vi "Get Root Elements.vi"(8 "error in (no error)":errorcluster, 11 "xml structure in":T1) -> (0 "error out":errorcluster, 1 "tag indices":i32[](array[numeric]), 2 "tag names":string[](array[string]), 3 "xml structure out":T1)   [LabVIEW 2011]
uses:
  XML Structure - Cluster.ctl
  XML Tag Type - Enum.ctl
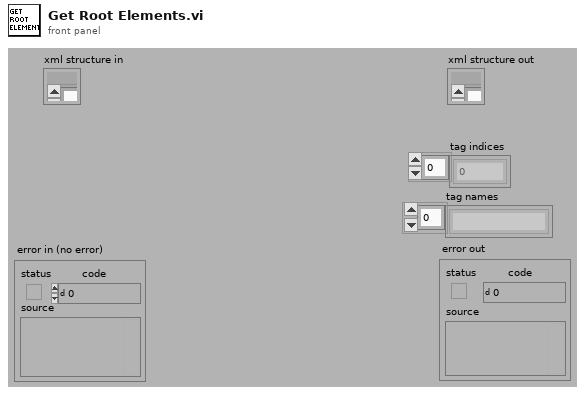
[diagram p1: front panel]
types:
  T1 = typedef "XML Structure - Cluster.ctl" = cluster{"tags":string[], "tag names":string[], "tag type":T2[], "offset":i32[], "close tag index":i32[], "xml":string, "Children":cluster{"children":i32[]}[], "parent index":i32[]}
  T2 = typedef "XML Tag Type - Enum.ctl" = enum16{"start tag", "empty tag", "end tag"}
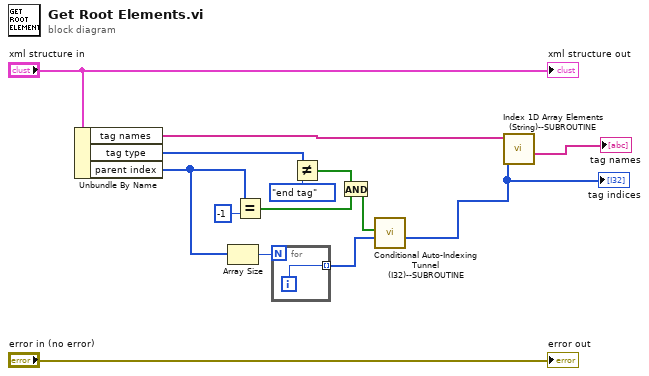
[diagram p0: block diagram]
diagram:
  n1 = Unbundle By Name("xml structure in") -> ("tag names"=w11:string[], "tag type"=w7:T2[], "parent index"=w2:i32[])
  n2 = Array Size(array=w2) -> (size(s)=w1:i32)
  n3 = Equal?(x=w2, y=-1) -> (x = y?=w4:bool[])
  n4 = for {
    N: w1 -> [_]
    tunnel: [w15] -> w9 mode=indexing
    i -> [w15]
  }
  n5 = Not Equal?(x=w7, y=XML_Tag_Type_-_Enum."end tag") -> (x != y?=w5:bool[])
  n6 = And(x=w5, y=w4) -> (x .and. y?=w3:bool[])
  n7 = call "Conditional Auto-Indexing Tunnel (I32)--SUBROUTINE.vi"("Array in"=w9, "Elements to keep"=w3) -> ("Filtered Array out"=w8:i32[])  [unwired: 5 in]
  "tag indices" <- w8
  n8 = call "Index 1D Array Elements (String)--SUBROUTINE.vi"("indices"=w8, "array"=w11) -> ("elements"=→"tag names":string[])  [unwired: 9 in]
  "xml structure out" <- "xml structure in"
  "error out" <- "error in (no error)"
